vi "buildClassFolder.vi"(9 "OldVal":string, 10 "NewVal":string, 11 "folder":path) -> (3 "appended path":path)   [LabVIEW 2023]
uses:
  <vilib>/Utility/error.llb/Trim Whitespace One-Sided.vi
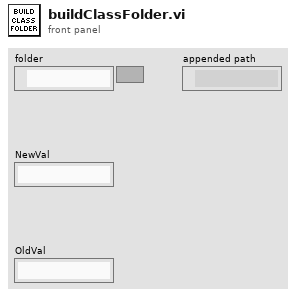
[diagram p1: front panel]
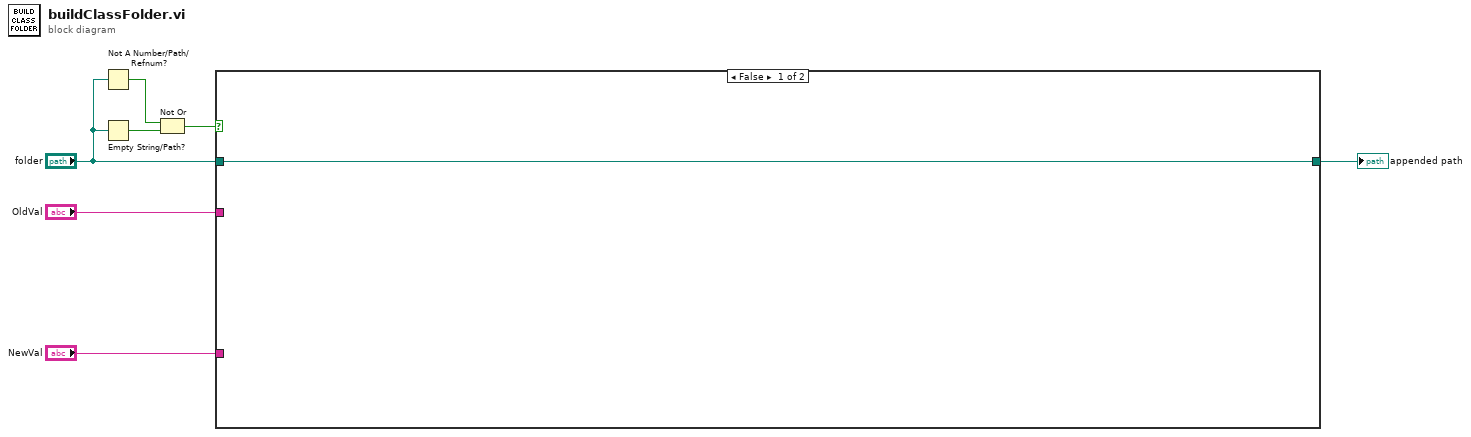
[diagram p0: block diagram]
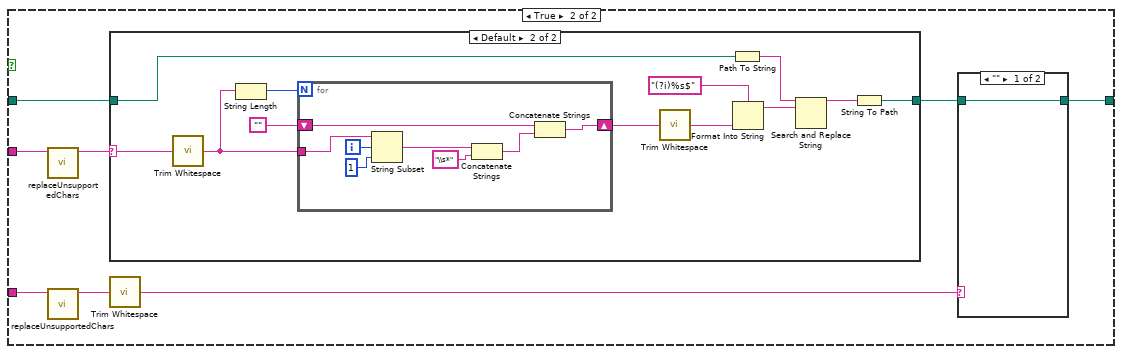
[diagram p2: hidden frame]
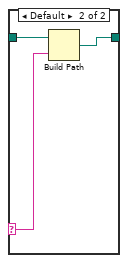
[diagram p3: hidden frame]
diagram:
  n1 = Not A Number/Path/Refnum?(number/path/refnum="folder") -> (NaN/Path/Refnum?=w5:bool)
  n2 = Empty String/Path?(string/path="folder") -> (empty?=w4:bool)
  n3 = Not Or(1:w4, 2:w5) -> (0:w2:bool)
  n4 = case shown="False" w2 {
    tunnel: [w8 w16] -> w7
    tunnel: "NewVal" -> [_ w12]
    tunnel: "folder" -> [w8 w11]
    tunnel: "OldVal" -> [_ w10]
    frame False {
    }
    frame True {
      n5 = call "replaceUnsupportedChars.vi"("stringIn"=w10) -> ("stringOut"=w9:string)  [unwired: 9 in, 1 out]
      n6 = call "replaceUnsupportedChars.vi"("stringIn"=w12) -> ("stringOut"=w13:string)  [unwired: 9 in, 1 out]
      n7 = case shown="Default" w9 {
        selector: w9 -> [_ w25]
        tunnel: [w21 w31] -> w14
        tunnel: w11 -> [w21 w30]
        frame "" {
        }
        frame Default {
          n8 = call <vilib>:"Trim Whitespace.vi"("string"=w25) -> ("trimmed string"=w22:string)  [unwired: 1 in]
          n9 = String Length(string=w22) -> (length=w28:i32)
          n10 = for {
            N: w28 -> [_]
            tunnel: w22 -> [w41]
            shift-right: [w38] -> w26
            shift-left: "" -> [w37]
            i -> [w40]
            n11 = String Subset(string=w41, offset (0)=w40, length (rest)=1 ("length (rest)")) -> (substring=w36:string)
            n12 = Concatenate Strings(w36, "\\s*" ("format string")) -> (w34:string)
            n13 = Concatenate Strings(w37, w34) -> (w38:string)
          }
          n14 = call <vilib>:"Trim Whitespace.vi"("string"=w26) -> ("trimmed string"=w24:string)  [unwired: 1 in]
          n15 = Path To String(path=w30) -> (string=w29:string)
          n16 = Format Into String(format string="(?i)%s$", w24) -> (resulting string=w23:string)  [unwired: 2 in, 1 out]
          n17 = Search and Replace String(input string=w29, search string=w23) -> (result string=w32:string)  [unwired: 6 in, 3 out]
          n18 = String To Path(string=w32) -> (path=w31:path)
        }
      }
      n19 = call <vilib>:"Trim Whitespace.vi"("string"=w13) -> ("trimmed string"=w15:string)  [unwired: 1 in]
      n20 = case shown="\"\"" w15 {
        selector: w15 -> [_ w20]
        tunnel: w14 -> [w17 w19]
        tunnel: [w17 w18] -> w16
        frame "" {
        }
        frame Default {
          n21 = Build Path(base path=w19, name or relative path=w20) -> (appended path=w18:path)
        }
      }
    }
  }
  "appended path" <- w7
